vi "Calib_global.vi"() -> ()   [LabVIEW 2013]
uses:
  Controls/TypeCalib.ctl
  Controls/Ref_Inst_type.ctl
  Controls/Cal_Inst_type.ctl
panel:
  out "Ch & Spans":T1[](array[typedef]) {"Ch No" min=0 max=7; "low limit (-10V)" min=-10 max=10 format="%.3f"; "high limit (10V)" min=-10 max=10 format="%.3f"}
  in  "ADAM Channel Name Vel Ref":string
  in  "Calib Ch No":string
  out "Temp (deg C)":dbl=21.0 format="%.1f"
  in  "Calib Raw Data Folder":path
  out "Instument setup Info":string
  out "Calibration Points":dbl[](array[numeric]) format="%.2f"
  in  "ADAM Channel Name":string
  in  "New Setup String":string
  in  "Pre Setup String":string
  in  "Calib file":path
  in  "Unmaned running":bool
  out "Instrument type":T2=enum."Hot wire"
  out "2nd ref instrument":T4={"2nd Ref type"=enum."Pitot-static tube", "2nd inst present"=FALSE}
  out "Ref velocity":dbl[](array[numeric]) format="%.3f"
  out "Ref Inst present":bool
  out "orig vel calib points":dbl[][](array[numeric]) format="%.2f"
  out "angle calib points":dbl[][](array[numeric]) format="%.2f"
  out "aux calib file string":string
  out "angle/vel Calib const":dbl[](array[numeric]) format="%.6f"
  out "Angle/vel calib file string":string="Title\tCross wire velocity calibration\rMethod \tThe Cross wire was calibrated for velocity against a Pitot-static tube.\rDate\t9/7/96\rTime\t10:59 am\rSeconds since 1/1/04\t2919754769\rFile name\tXWVE01-09/07/96\rCalib temp\t22.000000\rLab Pres\t1019.500000\rRef Inst calib file\tFCO16-24/10/95\rBoard type\tNB-MIO-16H\r\rChannel No 2\tCross wire 1\rOff Ch No\t1.000000\rOffset voltage\t3.198242\rGain\t8.000000\rPrecision mV\t0.610352\r\rChannel No 3\tCross wire 2\rOff Ch No\t1.000000\rOffset voltage\t3.198242\rGain\t8.000000\rPrecision mV\t0.610352\r\rChannel No 4\tMano \rOff Ch No\t0.000000\rOffset voltage\t0.498047\rGain\t8.000000\rPrecision mV\t0.610352\r\r\rCoeff n1\t0.535000\rCoeff A1\t7.693734\rCoeff B1\t3.274185\rAv % Err1\t0.079461\r\rCoeff n2\t0.540000\rCoeff A2\t7.248700\rCoeff B2\t3.147670\rAv % Err2\t0.156671\r\rBridge 1\tDISA 56 C16\rProbe type\tP51(Dual slant, plated)\rWire ID\t252\rOverheat ratio 1\t0.760000\rGain 1\t2.000000\rLP Filter Hz 1\t3000.000000\r\rBridge 2\tDISA 56 C16\rProbe type\tP51(Dual slant, plated)\rWire ID\t252\rOverheat ratio 2\t0.760000\rGain 2\t2.000000\rLP Filter Hz 2\t3000.000000\rCalib points label Start\r\rVelocity m/s\tVoltage1\tVoltage2\t\tEOH\r2.1926124347E+0\t3.5606311035E+0\t3.4721389160E+0\t0.0000000000E+0\t\r2.0274876172E+0\t3.5314160156E+0\t3.4438962402E+0\t0.0000000000E+0\t\r1.5937623952E+0\t3.4492885742E+0\t3.3619211426E+0\t0.0000000000E+0\t\r1.3049427194E+0\t3.3862644043E+0\t3.2982739258E+0\t0.0000000000E+0\t\r9.7343924857E-1\t3.3114423828E+0\t3.2225231934E+0\t0.0000000000E+0\tnot included\r6.0120920631E-1\t3.1918801270E+0\t3.1049123535E+0\t0.0000000000E+0\t\r4.5218630740E-1\t3.0609221191E+0\t2.9760163574E+0\t0.0000000000E+0\tnot included\r4.5464416266E-1\t3.0501985677E+0\t2.9740592448E+0\t0.0000000000E+0\tnot included\rEOD\r\r\rCalib points label End\r\r"
  out "existing angle calib":bool=TRUE
  out "Angle/vel calib file":path
  out "calib units":string
  out "Ref Instrument type":T3=enum."Enter Value"
  out "Header string":string="HW calib label Start\rTitle\tHot wire velocity calibration\rMethod \tThe Hot wire was calibrated for velocity against the LDA.\rDate\t29/7/97\rTime\t10:00\rSeconds since 1/1/04\t2953015250\rFile name\tsw36/29.7.97\rCalib temp\t25.000000\rLab Pres\t1022.000000\rBoard type\tNB-MIO-16H\r\rChannel No 1\tHW\rOff Ch No\t1.000000\rOffset voltage\t3.999023\rGain\t8.000000\rPrecision mV\t0.610352\r\r\rCoeff n\t0.405000\rCoeff A\t7.730378\rCoeff B\t6.204067\rAv % Err\t0.204301\r\rBridge\tPSI 6110\rProbe type\tP05 (Boundary, plated)\rWire ID\t159\rOverheat ratio\t0.700000\rGain\t1.000000\rLP Filter Hz\t1000.000000\rCalib points label Start\r\rVelocity m/s\tVoltage\t\tEOH\r9.5564835727E-1\t3.7365238525E+0\t0.0000000000E+0\t0.0000000000E+0\tnot included\r6.5982181910E-1\t3.6015061049E+0\t0.0000000000E+0\t0.0000000000E+0\t\r7.7799752697E-1\t3.6515397528E+0\t0.0000000000E+0\t0.0000000000E+0\tnot included\r7.8446760896E-1\t3.6542069285E+0\t0.0000000000E+0\t0.0000000000E+0\t\r1.0323890921E+0\t3.7452332047E+0\t0.0000000000E+0\t0.0000000000E+0\t\r1.2439956251E+0\t3.8077872140E+0\t0.0000000000E+0\t0.0000000000E+0\t\r1.6390568156E+0\t3.9125429351E+0\t0.0000000000E+0\t0.0000000000E+0\t\r2.1064482009E+0\t4.0145836958E+0\t0.0000000000E+0\t0.0000000000E+0\t\r2.6205967452E+0\t4.1107519190E+0\t0.0000000000E+0\t0.0000000000E+0\t\rEOD\r\r\rCalib points label End\r\r\rHW calib label End\r\r"
  out "Ref calib file string":string="Mano calib label Start\rTitle\tMicro manometer pressure calibration\rMethod \tThe Micro manometer was calibrated against the reading entered by the user.\rDate\t30/6/97\rTime\t16:10\rSeconds since 1/1/04\t2950531827\rFile name\tmano1/30.7.97\rCalib temp\t23.000000\rLab Pres\t1000.000000\rBoard type\tNB-MIO-16H\r\rChannel No 4\tMano \rOff Ch No\t0.000000\rOffset voltage\t0.996094\rGain\t8.000000\rPrecision mV\t0.610352\r\r\rCoeff A\t-0.006734\rCoeff B\t2.499596\rAv % Err\t0.327819\rManual zeroing\r0- 20 mmH20 range\rCalib points label Start\r\rPressure mmH2O\tVoltage\t\tEOH\r7.1000000000E-2\t1.6910461426E-1\t0.0000000000E+0\t0.0000000000E+0\t\r1.3300000000E-1\t3.2580078125E-1\t0.0000000000E+0\t0.0000000000E+0\t\r2.2900000000E-1\t5.6531188965E-1\t0.0000000000E+0\t0.0000000000E+0\t\r5.4000000000E-1\t1.3483123779E+0\t0.0000000000E+0\t0.0000000000E+0\t\r9.8700000000E-1\t2.2454833984E+0\t0.0000000000E+0\t0.0000000000E+0\tnot included\r7.9100000000E-1\t1.9670898437E+0\t0.0000000000E+0\t0.0000000000E+0\t\rEOD\r\r\rCalib points label End\r\r\rMano calib label End\r\r"
  out "Abs Press (mbar)":dbl=1022.0 format="%.2f"
  out "Ref Calib const":dbl[](array[numeric])=[-0.006734, 2.499596] format="%.6f"
  in  "Ref Calib file":path
  # "A              B"
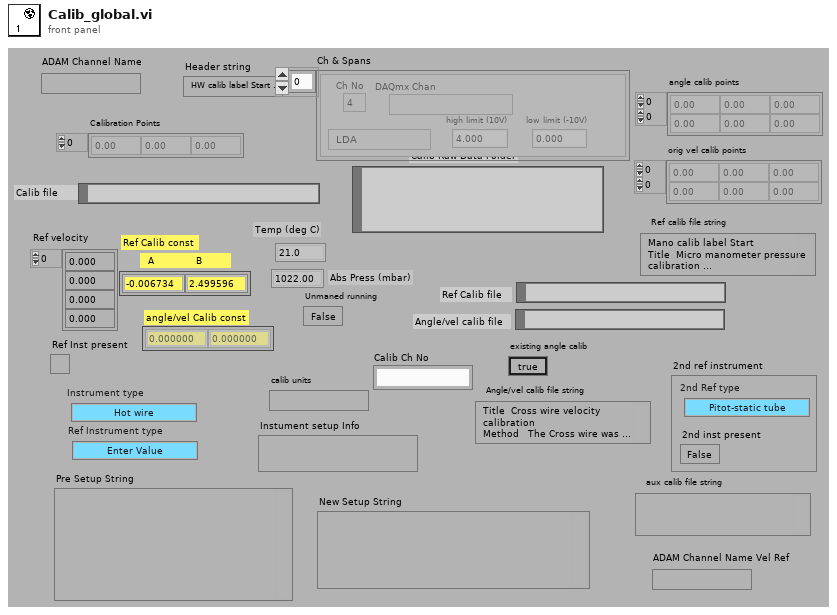
[diagram p1: front panel]
types:
  T1 = typedef "TypeCalib.ctl" = cluster{"high limit (10V)":sgl, "low limit (-10V)":sgl, "Ch No":i16, "Var name":string, "DAQmx Chan":tag}
  T2 = typedef "Cal_Inst_type.ctl" = enum16{"Propeller anemometer", "Pressure Transducer", "Hot wire", "Cross wire velocity", "Cross wire angle", "Generic Linear", "Generic Polynomial", "Generic BackPoly", "Fast FID", "Thermocouple", "Cold wire", "Pulsed Wire"}
  T3 = typedef "Ref_Inst_type.ctl" = enum16{"Propellor anemometer", "Pressure Transducer", "Raw voltage", "Pitot-static tube", "Preston tube", "Generic Linear", "Generic Polynomial", "Thermocouple", "LDA", "Enter Value", "ADAM Channel"}
  T4 = cluster{"2nd Ref type":T3, "2nd inst present":bool}
diagram:
